vi "StandAlone_TransientDataRead.vi"() -> ()   [LabVIEW 2019]
uses:
  <vilib>/Utility/file.llb/Read Delimited Spreadsheet (string).vi
  <vilib>/regexp/Match Regular Expression.xnode
panel:
  out "error out 2":errorcluster
  in  "Only OscilloscopeParamters_Total.csv, SampleData, SamplePerCap, and Waveform Data?":bool
  in  "Number of non-cap files":i32
  out "all rows":string[][](array[string])
  in  "base path":path=path "C:/Users/Aerolab1/Documents/LabVIEW Data/2019(64-bit)/Projects/SandboxOutputs"
  in  "run number":string
  out "Sets of Files":i32
  out "Total Files":i32
  out "file path (use dialog)":path=path "C:/Users/Aerolab1/Documents/LabVIEW Data/2019(64-bit)/Projects/GeneralSubVI/Outputs/Report/DataCollection_lightV16/run_2"
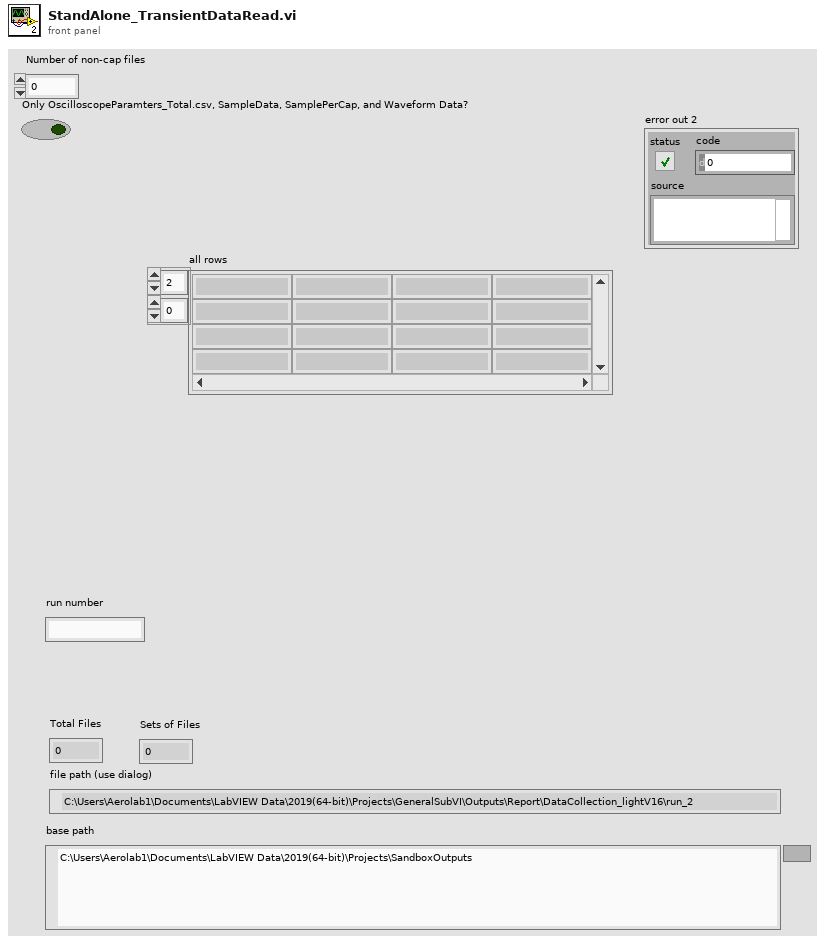
[diagram p1: front panel]
types:
  T1 = cluster{"created path":path, "created path":path}
  T2 = enum16{"big-endian, network order", "native, host order", "little-endian"}
  T3 = enum16{"open", "replace", "create", "open or create", "replace or create", "replace or create with confirmation"}
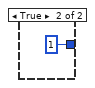
[diagram p4: hidden frame]
diagram:
  (unwired) 0.0
  (unwired) 3 ("y")
  # "Reused for laser scans in 2025 for the LT8650S March"
  # "Currently 1 though. need to make it 2 again"
  # "C:\\Users\\Aerolab1\\Documents\\LabVIEW Data\\2019(64-bit)\\Projects\\V2_General_Campaign_Filepath_Copy_Rename\\PART_Rename"
  # "C:\\Users\\Aerolab1\\Documents\\LabVIEW Data\\2019(64-bit)\\Projects\\Massachusetts2024\\RFBFIC\\BFICDATA"
  # "Decrementing bc one oscope parameters file and \nthe Forced Reset Timing .csv file"
  # "Number of file types\n1. Waveform Data \n2. SamplePerCap\n3. SampleData"
  n1 = Concatenate Strings("run_" ("string"), "run number") -> (w29:string)
  n2 = Build Path(base path="base path", name or relative path=w29) -> (appended path=w28:path)
  n3 = File/Directory Info(path=w28) -> (path out=w27:path)  [unwired: 1 in, 6 out]
  "file path (use dialog)" <- w27
  n4 = List Folder(path=w27) -> (filenames=w23:string[])  [unwired: 3 in, 3 out]
  n5 = case shown="False" "Only OscilloscopeParamters_Total.csv, SampleData, SamplePerCap, and Waveform Data?" {
    tunnel: w23 -> [w38 _]
    tunnel: [w34 1] -> w22
    frame False {
      n6 = for {
        tunnel: w38 -> [w45] mode=indexing
        shift-right: [w42] -> w36
        shift-left: 0 -> [w43]
        n7 = xnode "Match Regular Expression"("input string"=w45, "regular expression"="cap") -> ("offset past match"=w39:i32)  [unwired: 4 in, 4 out]
        n8 = Not Equal?(x=w39, y=-1) -> (x != y?=w41:bool)
        n9 = case shown="True" w41 {
          tunnel: w43 -> [w46 w48]
          tunnel: [w46 w47] -> w42
          frame False {
          }
          frame True {
            n10 = Increment(x=w48) -> (x+1=w47:i32)
          }
        }
      }
      n11 = Add(x=w36, y="Number of non-cap files") -> (x+y=w34:i32)
    }
    frame True {
    }
  }
  n12 = Build Path(base path=w27, name or relative path="Processed") -> (appended path=w31:path)
  n13 = Create Folder(path (use dialog)=w31) -> (created path=w4:path, error out=w20:errorcluster)  [unwired: 2 in, 1 out]
  n14 = Build Path(base path=w4, name or relative path="SupplementalNode") -> (appended path=w17:path)
  n15 = Build Path(base path=w4, name or relative path="DataNode") -> (appended path=w16:path)
  n16 = Array Size(array=w23) -> (size(s)=w26:i32)
  "Total Files" <- w26
  n17 = Subtract(x=w26, y=w22) -> (x-y=w25:i32)
  n18 = Create Folder(path (use dialog)=w17, error in=w20) -> (created path=w13:path, error out=w19:errorcluster)  [unwired: 1 in, 1 out]
  n19 = Quotient & Remainder(x=w25, y=3) -> (floor(x/y)=w1:i32)  [unwired: 1 out]
  "Sets of Files" <- w1
  n20 = Create Folder(path (use dialog)=w16, error in=w19) -> (created path=w12:path, error out=w18:errorcluster)  [unwired: 1 in, 1 out]
  n21 = Bundle("created path"=w12, "created path"=w13) -> (w11:T1)  [unwired: 1 in]
  n22 = for {
    N: w1 -> [_]
    tunnel: w27 -> [w173]
    tunnel: w11 -> [w172]
    shift-right: [w171] -> w7
    shift-left: w18 -> [w169]
    tunnel: [w164] -> w10
    i -> [w168]
    n23 = Increment(x=w168) -> (x+1=w170:i32)
    n24 = flat-sequence {
      tunnel: [w220] -> w189
      tunnel: [w219] -> w188
      tunnel: [""] -> w187
      tunnel: [w218] -> w186
      tunnel: [w214] -> w185
      tunnel: [w197] -> w184
      tunnel: w170 -> [w200]
      tunnel: [w199] -> w183
      tunnel: w173 -> [w198]
      tunnel: w172 -> [w197]
      tunnel: w169 -> [w196]
      tunnel: [w190] -> w167
      tunnel: w189 -> [w270]
      tunnel: w188 -> [w257]
      tunnel: w187 -> [w287]
      tunnel: w186 -> [w285]
      tunnel: [w286] -> w182
      tunnel: [w257] -> w181
      tunnel: [w285] -> w180
      tunnel: [w270] -> w179
      tunnel: [w262] -> w178
      tunnel: w185 -> [w284]
      tunnel: [w284] -> w177
      tunnel: w184 -> [w283]
      tunnel: [w283] -> w176
      tunnel: [w274] -> w175
      tunnel: [w282] -> w174
      tunnel: w183 -> [w282]
      tunnel: w167 -> [w263]
      tunnel: [w258] -> w166
      tunnel: [w259] -> w165
      tunnel: w182 -> [w334]
      tunnel: w181 -> [w335]
      tunnel: w180 -> [w333]
      tunnel: w179 -> [w332]
      tunnel: w178 -> [w331]
      tunnel: w177 -> [w330]
      tunnel: w176 -> [w325]
      tunnel: w175 -> [w322]
      tunnel: [w329] -> w171
      tunnel: w174 -> [w328]
      tunnel: w166 -> [w327]
      tunnel: w165 -> [w326]
      tunnel: [w322] -> w164
      frame #0 {
        (unwired) ""
        (unwired) i32[][] []
        (unwired) i32[][] []
        n25 = Number To Decimal String(number=w200) -> (decimal integer string=w199:string)  [unwired: 1 in]
        n26 = Concatenate Strings("SamplePerCap_" ("string"), w199, ".sbdf" ("string")) -> (w213:string)
        n27 = Concatenate Strings("SampleData_" ("string"), w199, ".sbdf" ("string")) -> (w210:string)
        n28 = Concatenate Strings("WaveformData_" ("string"), w199, ".sbdf" ("string")) -> (w207:string)
        n29 = Build Path(base path=w198, name or relative path=w213) -> (appended path=w202:path)
        n30 = Build Path(base path=w198, name or relative path=w210) -> (appended path=w203:path)
        n31 = Build Path(base path=w198, name or relative path="OscilloscopeParameters_Total.csv") -> (appended path=w195:path)
        n32 = Build Path(base path=w198, name or relative path=w207) -> (appended path=w201:path)
        n33 = call-poly <vilib>:"Read Delimited Spreadsheet.vi"("file path (dialog if empty)"=w195, "format (%s)"="%s", "delimiter (\\t)"="," ("delimiter (\\t)")) -> ("all rows"=w190:string[][], "error out"=w193:errorcluster)  [unwired: 7 in, 4 out]
        n34 = Open/Create/Replace File(file path (use dialog)=w201, operation (0:open)=T3."open", access (0:read/write)=enum16{"read/write", "read-only", "write-only"}."read-only") -> (refnum out=w240:refnum<file>, error out=w239:errorcluster)  [unwired: 3 in, 1 out]
        n35 = Open/Create/Replace File(file path (use dialog)=w202, operation (0:open)=T3."open", access (0:read/write)=enum16{"read/write", "read-only", "write-only"}."read-only") -> (refnum out=w228:refnum<file>, error out=w227:errorcluster)  [unwired: 3 in, 1 out]
        n36 = Open/Create/Replace File(file path (use dialog)=w203, operation (0:open)=T3."open", access (0:read/write)=enum16{"read/write", "read-only", "write-only"}."read-only") -> (refnum out=w252:refnum<file>, error out=w251:errorcluster)  [unwired: 3 in, 1 out]
        n37 = Set File Position(refnum=w240, from (0:start)=enum16{"start", "end", "current"}."start", error in=w239) -> (refnum out=w241:refnum<file>, error out=w242:errorcluster)  [unwired: 1 in]
        n38 = Set File Position(refnum=w228, from (0:start)=enum16{"start", "end", "current"}."start", error in=w227) -> (refnum out=w229:refnum<file>, error out=w230:errorcluster)  [unwired: 1 in]
        n39 = Set File Position(refnum=w252, from (0:start)=enum16{"start", "end", "current"}."start", error in=w251) -> (refnum out=w253:refnum<file>, error out=w254:errorcluster)  [unwired: 1 in]
        n40 = Read from Binary File(5:0.0, 8:w242, 9:T2."little-endian" ("byte order (0:big-endian, network order)"), 10:-1 ("count (1)"), 11:w241) -> (0:w244:errorcluster, 2:w220:dbl[], 3:w243:refnum<file>)  [unwired: 1 in, 1 out]
        n41 = Read from Binary File(5:0, 8:w230, 9:T2."little-endian" ("byte order (0:big-endian, network order)"), 10:-1 ("count (1)"), 11:w229) -> (0:w232:errorcluster, 2:w219:i32[], 3:w231:refnum<file>)  [unwired: 1 in, 1 out]
        n42 = Read from Binary File(5:i16 0, 8:w254, 9:T2."little-endian" ("byte order (0:big-endian, network order)"), 10:-1 ("count (1)"), 11:w253) -> (0:w256:errorcluster, 2:w218:i16[], 3:w255:refnum<file>)  [unwired: 1 in, 1 out]
        n43 = Close File(refnum=w243, error in=w244) -> (error out=w215:errorcluster)  [unwired: 1 out]
        n44 = Close File(refnum=w231, error in=w232) -> (error out=w217:errorcluster)  [unwired: 1 out]
        n45 = Close File(refnum=w255, error in=w256) -> (error out=w216:errorcluster)  [unwired: 1 out]
        n46 = Merge Errors(w196, w217, w216, w215, w193) -> (w214:errorcluster)
      }
      frame #1 {
        # "OFFSET"
        # "GAIN"
        # "May need to change"
        # "num_chan"
        # "num_iterations"
        # "gain"
        # "offset"
        # "xinc"
        # "num samples"
        n47 = Search/Split String(string=w287, search string/char (-)="datapoints_per_capture:") -> (match + rest of string=w314:string)  [unwired: 1 in, 2 out]
        n48 = Search/Split String(string=w314, search string/char (-)=":") -> (match + rest of string=w278:string)  [unwired: 1 in, 2 out]
        n49 = Scan String For Tokens(7:string[] ["%f"] ("operators (none)"), 8:1 ("offset"), 9:w278) -> (2:w308:i32)  [unwired: 3 in, 3 out]
        n50 = Add(x=13, y=w308) -> (x+y=w306:i32)
        n51 = Scan String For Tokens(7:string[] ["%f"] ("operators (none)"), 8:w306, 9:w278) -> (2:w305:i32)  [unwired: 3 in, 3 out]
        n52 = Add(x=w305, y=9) -> (x+y=w304:i32)
        n53 = Scan String For Tokens(7:string[] ["%.12f"] ("operators (none)"), 8:w304, 9:w278) -> (2:w301:i32)  [unwired: 3 in, 3 out]
        n54 = Add(x=w301, y=5) -> (x+y=w299:i32)
        n55 = Array Size(array=w257) -> (size(s)=w286:i32)
        n56 = Scan String For Tokens(7:string[] ["%.12f"] ("operators (none)"), 8:w299, 9:w278) -> (1:w290:string, 2:w297:i32)  [unwired: 3 in, 2 out]
        n57 = Search/Split String(string=w290, search string/char (-)=",") -> ()  [unwired: 1 in, 3 out]
        n58 = Add(x=w297, y=15 ("offset")) -> (x+y=w294:i32)
        n59 = Scan String For Tokens(7:string[] ["%f"] ("operators (none)"), 8:w294, 9:w278) -> (2:w291:i32)  [unwired: 3 in, 3 out]
        n60 = Add(x=w291, y=11 ("offset")) -> (x+y=w293:i32)
        n61 = Scan String For Tokens(7:string[] ["%f"] ("operators (none)"), 8:w293, 9:w278) -> (2:w281:i32)  [unwired: 3 in, 3 out]
        n62 = Add(x=w281, y=7) -> (x+y=w279:i32)
        n63 = Index Array(array=w263, index (row)=1, index (col)=1 ("disabled index (col)")) -> (element=w277:string)
        n64 = Decimal String To Number(string=w277, default (0L)=16 ("default (0 I32)")) -> (number=w262:i32)  [unwired: 1 in, 1 out]
        n65 = for {
          N: w262 -> [_]
          tunnel: w278 -> [w321]
          tunnel: [w319] -> _ mode=indexing
          shift-right: [w316] -> _
          shift-left: w279 -> [w318]
          n66 = Scan String For Tokens(7:string[] ["%d"] ("operators (none)"), 8:w318, 9:w321) -> (1:w319:string)  [unwired: 3 in, 3 out]
          n67 = Add(x=w318, y=2) -> (x+y=w316:i32)
        }
        n68 = Array Subset(array=w263, index (row)=2 ("index"), length (row)=w262, index (col)=1 ("index"), length (col)=1 ("length")) -> (w260:string[][])
        n69 = Array Subset(array=w263, index (row)=2 ("index"), length (row)=w262, index (col)=2 ("index"), length (col)=1 ("length")) -> (w261:string[][])
        n70 = Fract/Exp String To Number(string=w261) -> (number=w259:dbl[][])  [unwired: 3 in, 1 out]
        n71 = Array Subset(array=w263, index (row)=2 ("index"), length (row)=w262, index (col)=0 ("index"), length (col)=1 ("length")) -> (w274:string[][])
        n72 = Fract/Exp String To Number(string=w260) -> (number=w258:dbl[][])  [unwired: 3 in, 1 out]
        "all rows" <- w263
      }
      frame #2 {
        # "Samples within each\ncapture"
        # "Sample\nData"
        # "Waveform Data"
        # "Number\nChannels"
        # "Index Marker"
        n73 = Unbundle(w325) -> ("created path"=w324:path, "created path"=w323:path)
        n74 = for {
          N: w331 -> [w378]
          tunnel: w335 -> [w383]
          tunnel: w334 -> [w382]
          tunnel: w333 -> [w381]
          tunnel: w332 -> [w380]
          tunnel: w322 -> [w346] mode=indexing
          shift-right: [w347] -> w329
          shift-left: w330 -> [w368]
          tunnel: w328 -> [w357]
          tunnel: w327 -> [w345] mode=indexing
          tunnel: w326 -> [w341] mode=indexing
          tunnel: w324 -> [w337]
          tunnel: w323 -> [w336]
          i -> [w377]
          w354 = "%.15f" ("format string")
          w371 = "%.15f" ("format string")
          # "Number of captures"
          n75 = Index Array(array=w341, index=0) -> (element=w340:dbl)
          n76 = Index Array(array=w345, index=0) -> (element=w343:dbl)
          n77 = for {
            N: w382 -> [_]
            tunnel: w383 -> [w389] mode=indexing
            tunnel: w381 -> [w435]
            tunnel: w380 -> [w438]
            tunnel: w377 -> [w434]
            tunnel: w378 -> [w428]
            shift-right: [w415] -> _
            shift-left: 0 -> [w437]
            tunnel: [w413] -> w339
            shift-right: [w408] -> _
            shift-left: dbl[][] [] ("array") -> [w409]
            shift-right: [w384] -> _
            shift-left: dbl[][] [] ("array") -> [w403]
            tunnel: [w384] -> w338
            tunnel: w343 -> [w385]
            tunnel: w340 -> [w386]
            i -> [w407]
            n78 = flat-sequence {
              tunnel: w389 -> [w472]
              tunnel: [w456] -> w439
              tunnel: w438 -> [w442]
              tunnel: w407 -> [w471]
              tunnel: w389 -> [w459]
              tunnel: w437 -> [w461]
              tunnel: [w465] -> w436
              tunnel: w435 -> [w465]
              tunnel: w434 -> [w463]
              tunnel: [w462] -> w433
              tunnel: [w461] -> w432
              tunnel: [w460] -> w429
              tunnel: w428 -> [w460]
              tunnel: [w459] -> w426
              tunnel: [w458] -> w424
              tunnel: [w447] -> w423
              tunnel: [w441] -> w421
              tunnel: [w440] -> w419
              tunnel: [w457] -> w410
              tunnel: w409 -> [w457]
              tunnel: [w455] -> w404
              tunnel: w403 -> [w455]
              tunnel: [w447] -> w398
              tunnel: [w446] -> w395
              tunnel: [w445] -> w393
              tunnel: [w444] -> w391
              tunnel: [w443] -> w390
              tunnel: w389 -> [w443]
              tunnel: w386 -> [w441]
              tunnel: w385 -> [w440]
              tunnel: w439 -> [w489]
              tunnel: w436 -> [w492]
              tunnel: w433 -> [w493]
              tunnel: w432 -> [w495]
              tunnel: [w495] -> w431
              tunnel: [w494] -> w430
              tunnel: w429 -> [w494]
              tunnel: [w491] -> w427
              tunnel: w426 -> [w491]
              tunnel: [w487] -> w425
              tunnel: w424 -> [w490]
              tunnel: w423 -> [w488]
              tunnel: [w485] -> w422
              tunnel: w421 -> [w485]
              tunnel: [w484] -> w420
              tunnel: w419 -> [w484]
              tunnel: [w483] -> w417
              tunnel: [w482] -> w411
              tunnel: w410 -> [w482]
              tunnel: [w480] -> w405
              tunnel: w404 -> [w480]
              tunnel: [w479] -> w399
              tunnel: w398 -> [w479]
              tunnel: [w478] -> w396
              tunnel: w395 -> [w478]
              tunnel: [w477] -> w394
              tunnel: w393 -> [w477]
              tunnel: [w476] -> w392
              tunnel: w391 -> [w476]
              tunnel: w390 -> [w475]
              tunnel: [w475] -> w388
              tunnel: w431 -> [w512]
              tunnel: w430 -> [w514]
              tunnel: w427 -> [w515]
              tunnel: w425 -> [w511]
              tunnel: w422 -> [w505]
              tunnel: w420 -> [w506]
              tunnel: [w509] -> w418
              tunnel: w417 -> [w509]
              tunnel: [w508] -> w416
              tunnel: [w507] -> w414
              tunnel: [w504] -> w412
              tunnel: w411 -> [w504]
              tunnel: [w503] -> w406
              tunnel: w405 -> [w503]
              tunnel: [w501] -> w402
              tunnel: [w500] -> w401
              tunnel: [w499] -> w400
              tunnel: w399 -> [w502]
              tunnel: [w502] -> w397
              tunnel: w396 -> [w501]
              tunnel: w394 -> [w500]
              tunnel: w392 -> [w499]
              tunnel: w388 -> [w498]
              tunnel: [w496] -> w387
              tunnel: w416 -> [w529]
              tunnel: w418 -> [w530]
              tunnel: [w526] -> w415
              tunnel: w414 -> [w526]
              tunnel: [w524] -> w413
              tunnel: w412 -> [w525]
              tunnel: [w524] -> w408
              tunnel: w406 -> [w519]
              tunnel: w402 -> [w522]
              tunnel: w401 -> [w521]
              tunnel: w400 -> [w520]
              tunnel: [w517] -> w384
              tunnel: w397 -> [w523]
              tunnel: w387 -> [w516]
              frame #0 {
                # "7 may become the number of\nsamples per capture. But not for\nnow because there is fidelity and\nparallelization tradeoffs"
                # "0. AbsoluteInitialX\n1. Xincrement\n2. Offset\n3. Gain\n4. Beam On? (1 yes, 0 no)\n5. Index of Maximum\n6. Rolling Transient Counter"
                n79 = Multiply(x=w471, y=5) -> (x*y=w451:i32)
                n80 = Multiply(x=w459, y=w463) -> (x*y=w464:i32)
                n81 = for {
                  N: w472 -> [_]
                  tunnel: [w473] -> w456 mode=indexing
                  i -> [w474]
                  n82 = To Double Precision Float(number=w474) -> (double precision float=w473:dbl)
                }
                n83 = Add(x=0, y=w451) -> (x+y=w466:i32)
                n84 = Add(x=1, y=w451) -> (x+y=w467:i32)
                n85 = Add(x=2, y=w451) -> (x+y=w450:i32)
                n86 = Add(x=3, y=w451) -> (x+y=w449:i32)
                n87 = Add(x=4, y=w451) -> (x+y=w448:i32)
                n88 = Add(x=w461, y=w464) -> (x+y=w462:i32)
                n89 = Index Array(array=w442, index=w466) -> (element=w447:dbl)
                n90 = Index Array(array=w442, index=w467) -> (element=w458:dbl)
                n91 = Index Array(array=w442, index=w449) -> (element=w445:dbl)
                n92 = Index Array(array=w442, index=w448) -> (element=w444:dbl)
                n93 = Index Array(array=w442, index=w450) -> (element=w446:dbl)
              }
              frame #1 {
                # "You may ask, but when you hit the beam is on, some of the values in the capture will be before the \nchange. To which you may be correct. I say to you this: that's rough, buddy"
                n94 = Multiply(x=w489, y=w490) -> (x*y=w481:dbl[])
                n95 = Array Subset(array=w492, index=w493, length=w491) -> (w486:i16[])
                n96 = Add(x=w481, y=w488) -> (x+y=w483:dbl[])
                n97 = To Double Precision Float(number=w486) -> (double precision float=w487:dbl[])
              }
              frame #2 {
                n98 = Multiply(x=w514, y=w515) -> (x*y=w513:i32)
                n99 = To Double Precision Float(number=w498) -> (double precision float=w497:dbl)
                n100 = Multiply(x=w511, y=w505) -> (x*y=w510:dbl[])
                n101 = Add(x=w513, y=w512) -> (x+y=w507:i32)
                n102 = Round To Nearest(number=w497) -> (nearest integer value=w496:dbl)
                n103 = Add(x=w510, y=w506) -> (x+y=w508:dbl[])
              }
              frame #3 {
                n104 = Build Array(w530, w529) -> (w528:dbl[][])
                n105 = Build Array(w523, w522, w521, w520, w516) -> (w518:dbl[])
                n106 = Transpose 2D Array(2D array=w528) -> (transposed array=w527:dbl[][])
                n107 = Insert Into Array(array=w519, new element=w518) -> (w517:dbl[][])  [unwired: 2 in]
                n108 = Insert Into Array(array=w525, new element=w527) -> (w524:dbl[][])  [unwired: 2 in]
              }
            }
          }
          n109 = Array To Spreadsheet String(array=w339, 3:w371) -> (spreadsheet string=w373:string)  [unwired: 1 in]
          n110 = Concatenate Strings("DataFileNode_" ("string"), w357, "_" ("string"), w346, ".txt" ("string")) -> (w375:string)
          n111 = Spreadsheet String To Array(format string=w371, spreadsheet string=w373, array type (2D Dbl)=string[][] []) -> (array=w366:string[][])  [unwired: 1 in]
          n112 = Array To Spreadsheet String(array=w338, 3:w354) -> (spreadsheet string=w356:string)  [unwired: 1 in]
          n113 = Spreadsheet String To Array(format string=w354, spreadsheet string=w356, array type (2D Dbl)=string[][] []) -> (array=w351:string[][])  [unwired: 1 in]
          n114 = Concatenate Strings("SupplementalDataFileNode_" ("string"), w357, "_" ("string"), w346, ".txt" ("string")) -> (w358:string)
          n115 = Array To Spreadsheet String(delimiter (Tab)=",", array=w351, 3:"%s" ("format string")) -> (spreadsheet string=w349:string)
          n116 = Build Path(base path=w337, name or relative path=w375) -> (appended path=w367:path)
          n117 = Build Path(base path=w336, name or relative path=w358) -> (appended path=w350:path)
          n118 = Array To Spreadsheet String(delimiter (Tab)=",", array=w366, 3:"%s" ("format string")) -> (spreadsheet string=w365:string)
          n119 = Write to Text File(file (use dialog)=w367, text=w365, error in=w368) -> (error out=w348:errorcluster)  [unwired: 1 in, 2 out]
          n120 = Write to Text File(file (use dialog)=w350, text=w349, error in=w348) -> (error out=w347:errorcluster)  [unwired: 1 in, 2 out]
        }
      }
    }
  }
  n121 = Index Array(array=w10, index (col)=0 ("disabled index (col)")) -> (element=w8:string[])  [unwired: 1 in]
  n122 = Strip Path(path=w4) -> (stripped path=w3:path)  [unwired: 1 out]
  n123 = Strip Path(path=w3) -> (stripped path=w2:path)  [unwired: 1 out]
  n124 = disable-structure shown="Enabled" {
    disable-tunnel: w8 -> [w535 _]
    disable-tunnel: w7 -> [w534 _]
    disable-tunnel: w2 -> [w533 _]
    disable-tunnel: "run number" -> [w532 _]
    disable-tunnel: [w531 _] -> w5
    frame Enabled {
      n125 = call "ReadTextFiles2ExcelCSV_Subvi.vi"("error out"=w534, "Array"=w535, "Run Number"=w532, "base path"=w533) -> ("error out 2"=w531:errorcluster)  [unwired: 7 in]
    }
    frame Disabled {
    }
  }
  "error out 2" <- w5
  n126 = call <vilib>:"Simple Error Handler.vi"("error in (no error)"=w5) -> ()  [unwired: 4 in, 5 out]
